vi "Prober_LoadUnload.vi"(8 "error in (no error)":errorcluster, 11 "ProbeStationControl in":refnum<class "ProbeStationControl.lvclass">) -> (0 "error out":errorcluster, 2 "Home or Load?":enum16{"Home", "Load"}(ring), 3 "ProbeStationControl out":refnum<class "ProbeStationControl.lvclass">)   [LabVIEW 2013, in "ProbeStationControl.lvclass"]
uses:
  ProbeStationControl.lvclass
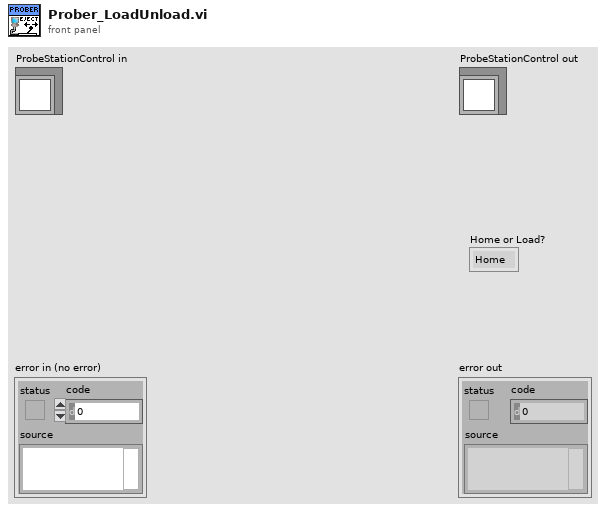
[diagram p1: front panel]
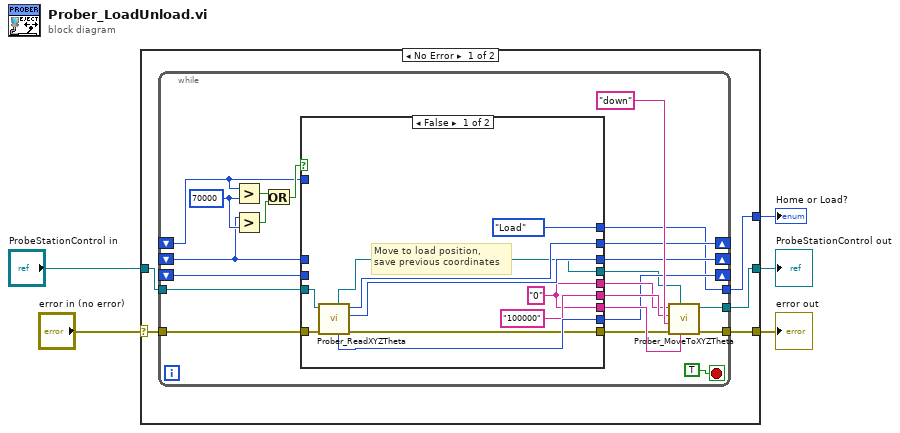
[diagram p0: block diagram]
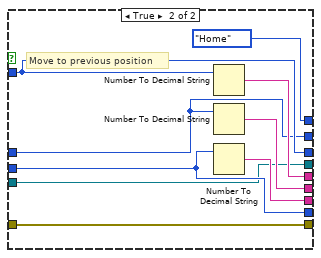
[diagram p2: hidden frame]
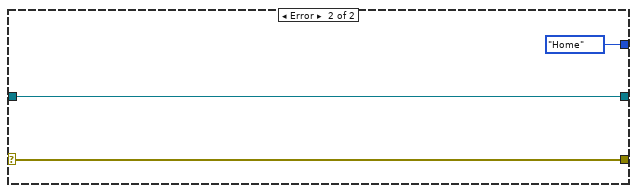
[diagram p3: hidden frame]
diagram:
  n1 = case shown="No Error" "error in (no error)" {
    selector: "error in (no error)" -> [w10 w54]
    tunnel: [w9 w54] -> w4
    tunnel: "ProbeStationControl in" -> [w6 w52]
    tunnel: [w8 enum16{"Home", "Load"}."Home" ("Home or Load?")] -> w3
    tunnel: [w7 w52] -> w1
    frame No Error {
      n2 = while {
        shift-right: [w20] -> _
        shift-left: _ -> [w27]
        shift-right: [w19] -> _
        shift-left: _ -> [w26]
        shift-right: [w18] -> _
        shift-left: _ -> [w25]
        tunnel: w10 -> [w16]
        tunnel: [w17] -> w9
        tunnel: [w14] -> w8
        tunnel: [w13] -> w7
        tunnel: w6 -> [w12]
        stop <- TRUE stop-if-true
        w29 = 70000 ("y")
        n3 = Greater?(x=w27, y=w29) -> (0:w32:bool)
        n4 = Greater?(x=w26, y=w29) -> (0:w31:bool)
        n5 = Or(x=w32, y=w31) -> (x .or. y?=w28:bool)
        n6 = case shown="False" w28 {
          tunnel: w27 -> [_ w48]
          tunnel: w26 -> [_ w47]
          tunnel: w25 -> [_ w46]
          tunnel: [w38 w51] -> w23
          tunnel: ["100000" w50] -> w22
          tunnel: [w38 w49] -> w21
          tunnel: [w42 w47] -> w20
          tunnel: [w41 w48] -> w19
          tunnel: [w40 w46] -> w18
          tunnel: w16 -> [w37 w45]
          tunnel: [w36 w45] -> w15
          tunnel: [enum16{"Home", "Load"}."Load" ("Home or Load?") enum16{"Home", "Load"}."Home" ("Home or Load?")] -> w14
          tunnel: w12 -> [w34 w43]
          tunnel: [w33 w43] -> w11
          frame False {
            w38 = "0"
            # "Move to load position,\nsave previous coordinates"
            n7 = call "Prober_ReadXYZTheta.vi"("error in (no error)"=w37, "ProbeStationControl in"=w34) -> ("error out"=w36:errorcluster, "Y location [µm]"=w41:i32, "X location [µm]"=w42:i32, "Theta location [mdeg]"=w40:i32, "ProbeStationControl out"=w33:refnum<class "ProbeStationControl.lvclass">)  [unwired: 4 in, 1 out]
          }
          frame True {
            # "Move to previous position"
            n8 = Number To Decimal String(number=w48) -> (decimal integer string=w49:string)  [unwired: 1 in]
            n9 = Number To Decimal String(number=w47) -> (decimal integer string=w50:string)  [unwired: 1 in]
            n10 = Number To Decimal String(number=w46) -> (decimal integer string=w51:string)  [unwired: 1 in]
          }
        }
        n11 = call "Prober_MoveToXYZTheta.vi"("Theta location [mdeg]"=w23, "ProbeStationControl in"=w11, "error in (no error)"=w15, "Z location [µm]"="down", "Y location [µm]"=w22, "X location [µm]"=w21) -> ("error out"=w17:errorcluster, "ProbeStationControl out"=w13:refnum<class "ProbeStationControl.lvclass">)  [unwired: 3 in, 1 out]
      }
    }
    frame Error {
    }
  }
  "error out" <- w4
  "Home or Load?" <- w3
  "ProbeStationControl out" <- w1
